vi "ALTERA_BAT.vi"(0 "file path (use dialog)":path, 5 "Diretório de trabalho (.atp)":string="C:\\Users\\Flavio-CPGEI\\Documents\\ATPdata\\work", 7 "Nome do arquivo":string, 9 "Diretório de saída":string="C:\\Users\\Flavio-CPGEI\\Documents\\simulacoes", 11 "error in":errorcluster, 12 "Diretório de saída (arquivos atp)":string="D:\\arquivos_atp") -> (4 "path":path, 15 "error out":errorcluster)   [LabVIEW 2020]
panel:
  out "concatenated string":string
  in  "Diretório runATP.exe  (NÃO USADO)":string="C:\\ATP\\tools"
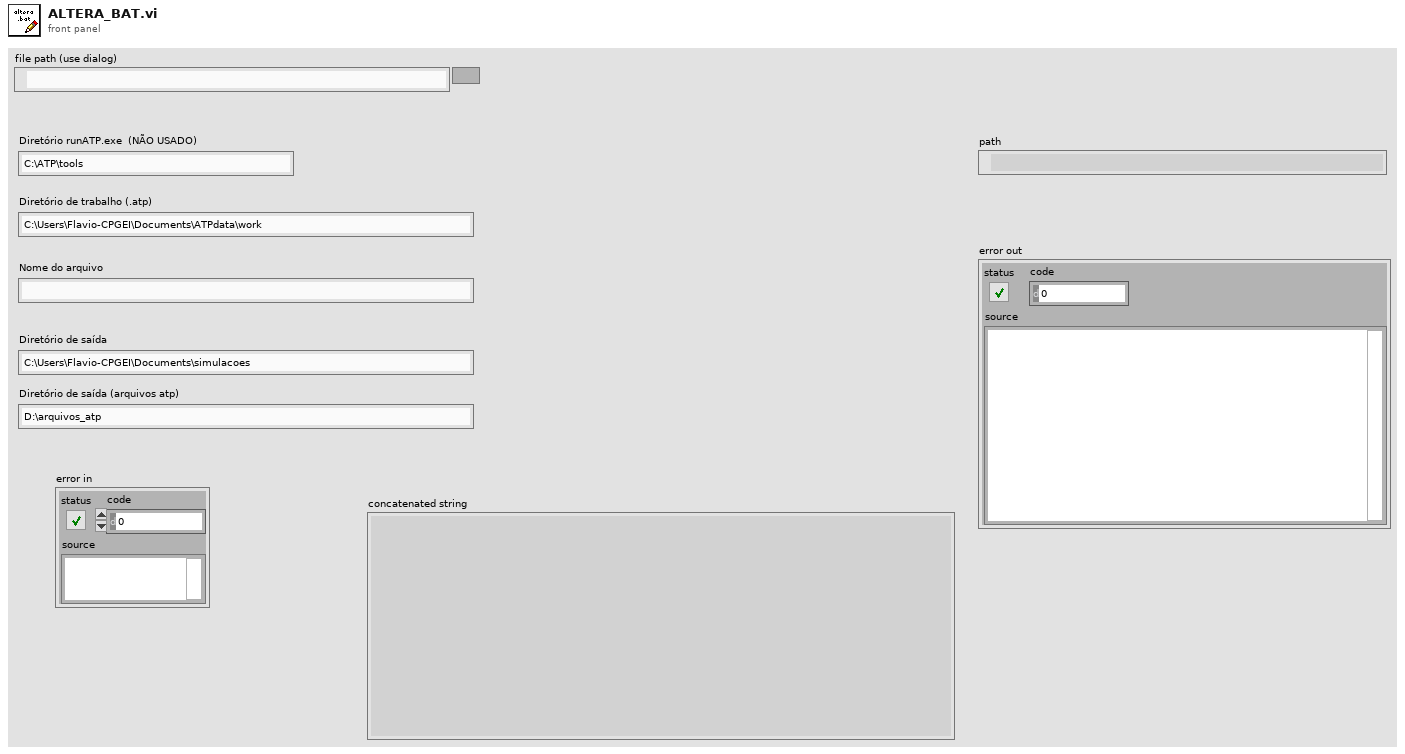
[diagram p1: front panel]
types:
  T1 = enum16{"open", "replace", "create", "open or create", "replace or create", "replace or create with confirmation"}
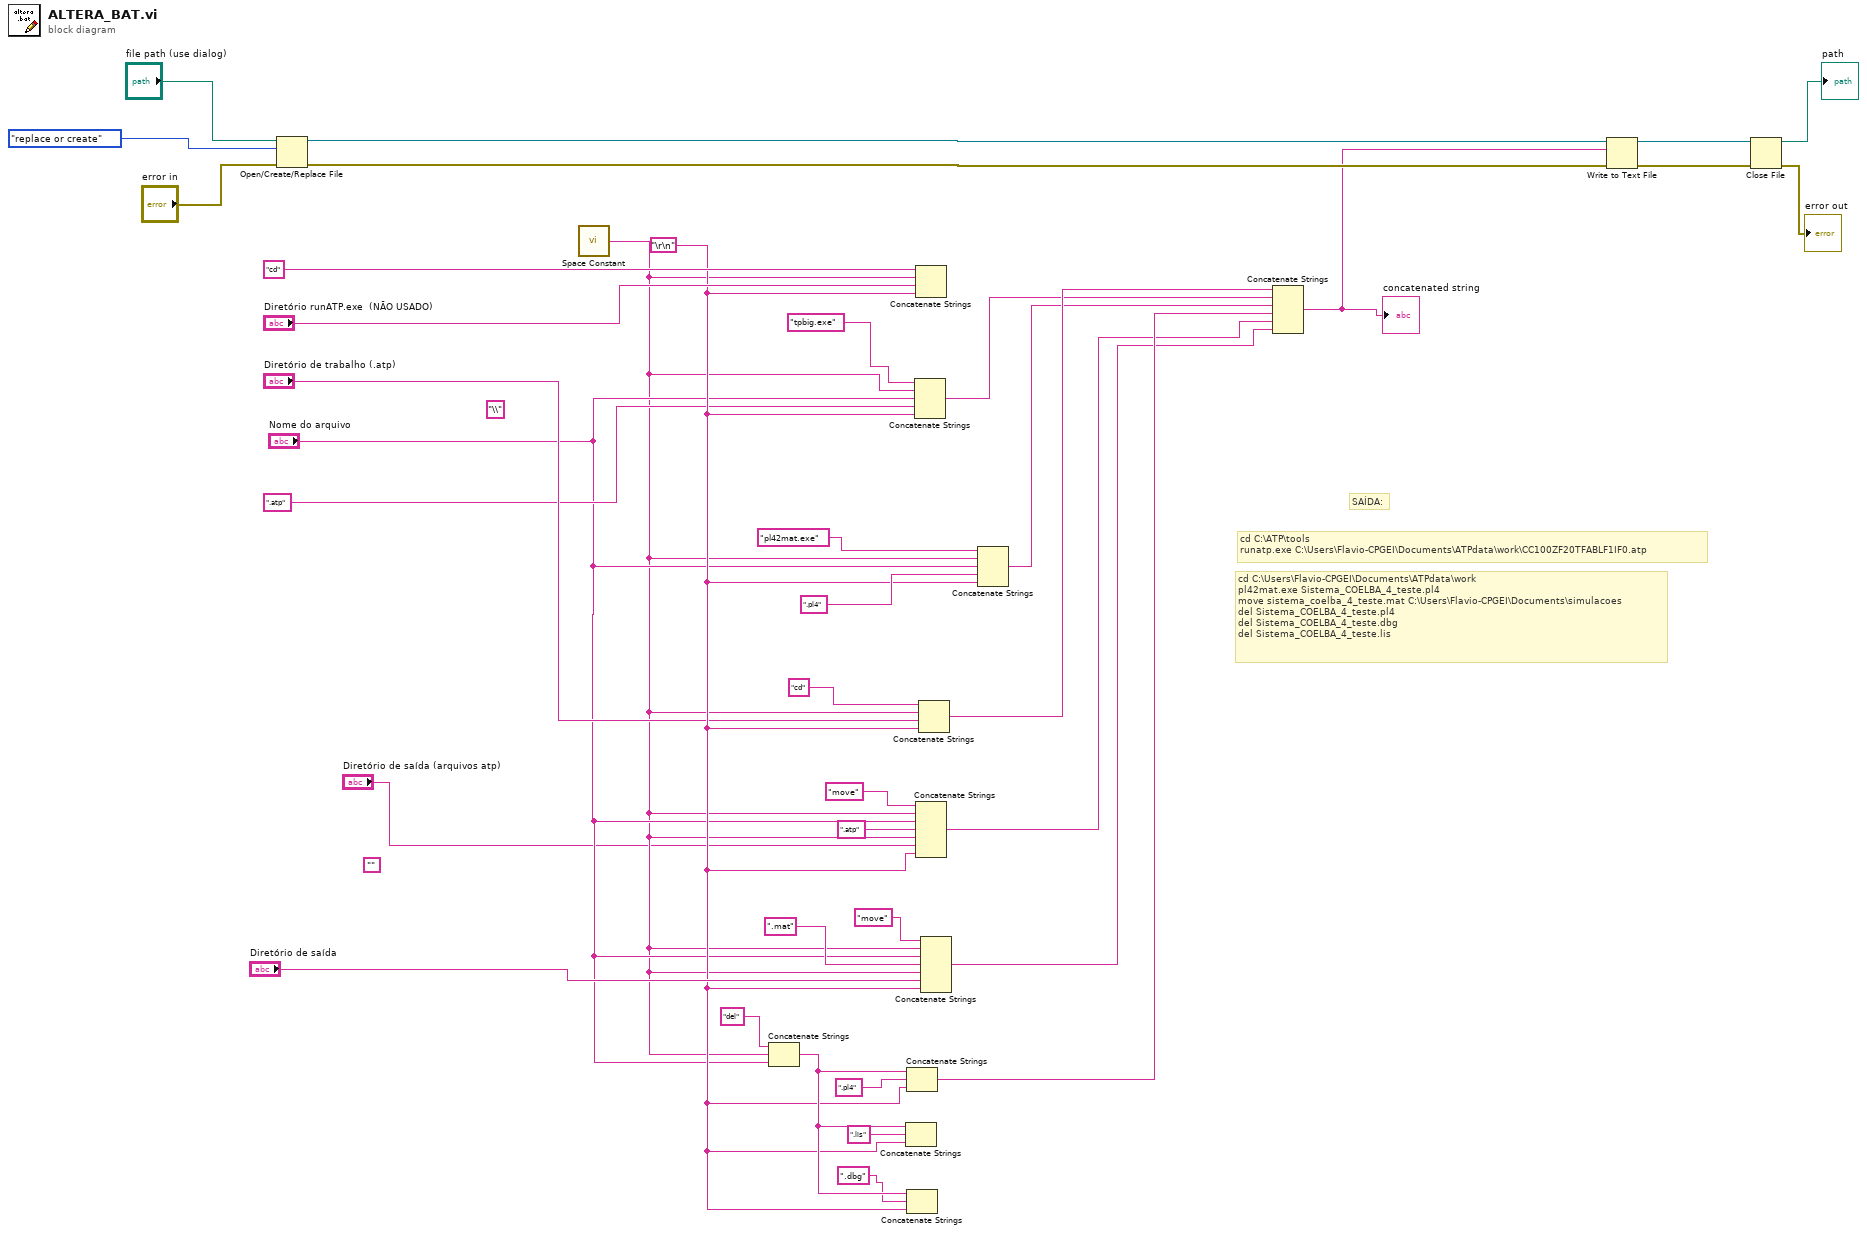
[diagram p0: block diagram]
diagram:
  (unwired) ""
  w13 = "\r\n"
  (unwired) "\\"
  # "SAÍDA:"
  # "cd C:\\ATP\\tools\nrunatp.exe C:\\Users\\Flavio-CPGEI\\Documents\\ATPdata\\work\\CC100ZF20TFABLF1IF0.atp"
  # "cd C:\\Users\\Flavio-CPGEI\\Documents\\ATPdata\\work\npl42mat.exe Sistema_COELBA_4_teste.pl4\nmove sistema_coelba_4_teste.mat C:\\Users\\Flavio-CPGEI\\Documents\\simulacoes\ndel Sistema_COELBA_4_teste.pl4\ndel Sistema_COELBA_4_teste.dbg\ndel Sistema_COELBA_4_teste.lis"
  n1 = Open/Create/Replace File(file path (use dialog)="file path (use dialog)", error in="error in", operation (0:open)=T1."replace or create") -> (refnum out=w36:refnum<file>, error out=w37:errorcluster)  [unwired: 3 in, 1 out]
  n2 = call <vilib>:"Space Constant.vi"() -> ("String"=w6:string)
  n3 = Concatenate Strings("del" ("string"), w6, "Nome do arquivo") -> (w16:string)
  n4 = Concatenate Strings(w16, ".lis" ("string"), w13) -> ()  [unwired: 1 out]
  n5 = Concatenate Strings(w16, ".pl4" ("string"), w13) -> (w4:string)
  n6 = Concatenate Strings(w16, ".dbg" ("string"), w13) -> ()  [unwired: 1 out]
  n7 = Concatenate Strings("tpbig.exe", w6, "Nome do arquivo", ".atp", w13) -> (w9:string)
  n8 = Concatenate Strings("cd", w6, "Diretório runATP.exe  (NÃO USADO)", w13) -> ()  [unwired: 1 out]
  n9 = Concatenate Strings("move" ("string"), w6, "Nome do arquivo", ".atp", w6, "Diretório de saída (arquivos atp)", w13) -> (w3:string)
  n10 = Concatenate Strings("cd", w6, "Diretório de trabalho (.atp)", w13) -> (w10:string)
  n11 = Concatenate Strings("move" ("string"), w6, "Nome do arquivo", ".mat" ("string"), w6, "Diretório de saída", w13) -> (w2:string)
  n12 = Concatenate Strings("pl42mat.exe" ("string"), w6, "Nome do arquivo", ".pl4", w13) -> (w8:string)
  n13 = Concatenate Strings(w10, w9, w8, w4, w3, w2) -> (w14:string)
  "concatenated string" <- w14
  n14 = Write to Text File(file (use dialog)=w36, text=w14, error in=w37) -> (refnum out=w34:refnum<file>, error out=w35:errorcluster)  [unwired: 1 in, 1 out]
  n15 = Close File(refnum=w34, error in=w35) -> (path=→"path":path, error out=→"error out":errorcluster)
